vi "String - Convert Str (YYYY-mm-dd HHcMMcSS) to TimeStamp.vi"(11 "YYYY-mm-dd HH:MM:SS (String)":string="2014-09-24 13:30:59") -> (2 "time stamp":timestamp format="%<%I:%M:%S%3u %p\n%x>T", 3 "YYYY-mm-dd HH:MM:SS (String)":string)   [LabVIEW 2013]
uses:
  <vilib>/Utility/miscctls.llb/LVDateTimeRec.ctl
panel:
  out ".fractional second":string
  out "SS":string
  out "MM":string
  out "HH":string
  out "dd":string
  out "mm":string
  out "YYYY":string
  out "YYYY-mm-dd":string
  out "HH:MM:SS":string
  out "Array":string[](array[string])
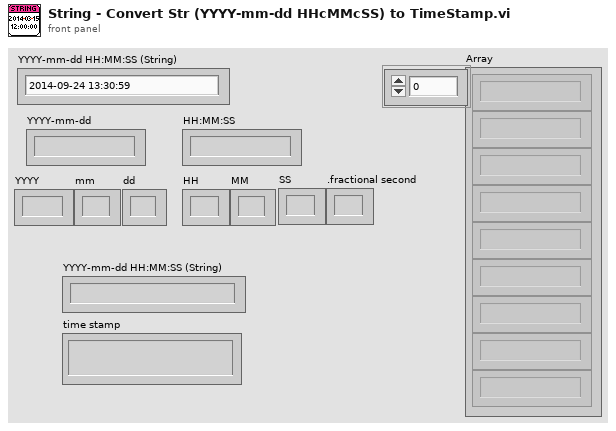
[diagram p1: front panel]
types:
  T1 = typedef "LVDateTimeRec.ctl" = cluster{"fractional second":dbl, "second":i32, "minute":i32, "hour":i32, "day of month":i32, "month":i32, "year":i32, "day of week":i32, "day of year":i32, "DST":i32}
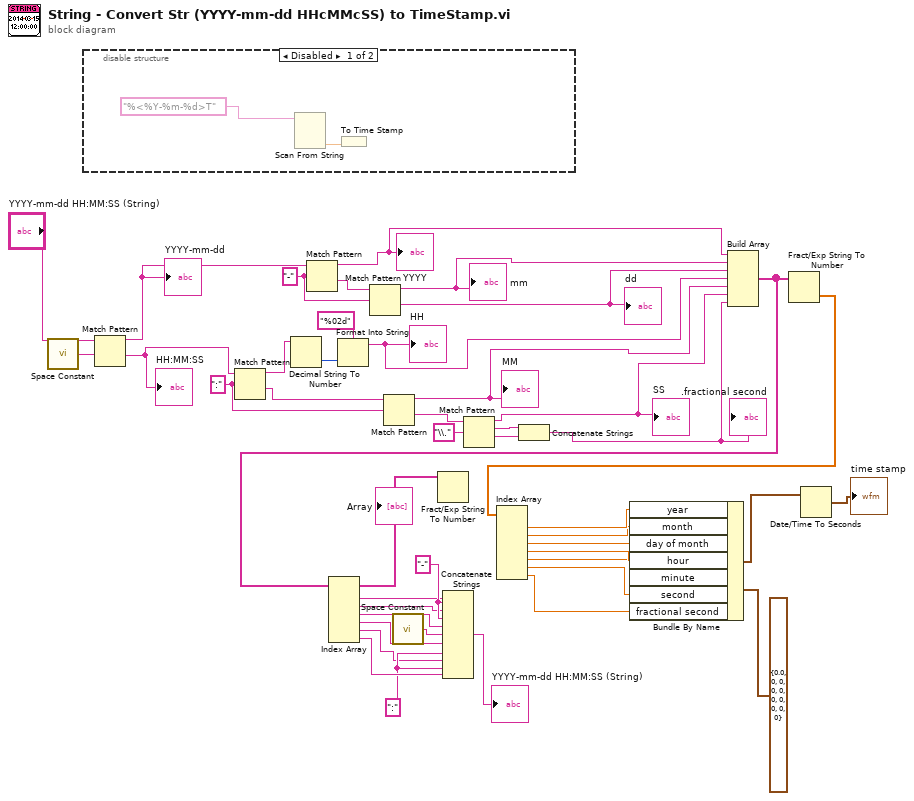
[diagram p0: block diagram]
diagram:
  w18 = ":" ("regular expression")
  w22 = "-" ("regular expression")
  w42 = ":"
  w38 = "-"
  n1 = call <vilib>:"Space Constant.vi"() -> ("String"=w24:string)
  n2 = disable-structure shown="Disabled" {
    frame Disabled {
      n3 = Scan From String(input string="%<%Y-%m-%d>T") -> (output 1=w45:dbl)  [unwired: 4 in, 3 out]
      n4 = To Time Stamp(1:w45) -> ()  [unwired: 1 out]
    }
    frame Enabled {
    }
  }
  n5 = Match Pattern(string="YYYY-mm-dd HH:MM:SS (String)", regular expression=w24) -> (before substring=w23:string, after substring=w20:string)  [unwired: 1 in, 2 out]
  "HH:MM:SS" <- w20
  "YYYY-mm-dd" <- w23
  n6 = Match Pattern(string=w20, regular expression=w18) -> (before substring=w3:string, after substring=w19:string)  [unwired: 1 in, 2 out]
  n7 = Decimal String To Number(string=w3) -> (number=w2:i32)  [unwired: 2 in, 1 out]
  n8 = Match Pattern(string=w23, regular expression=w22) -> (before substring=w17:string, after substring=w21:string)  [unwired: 1 in, 2 out]
  "YYYY" <- w17
  n9 = Format Into String(format string="%02d", w2) -> (resulting string=w1:string)  [unwired: 2 in, 1 out]
  "HH" <- w1
  n10 = Match Pattern(string=w21, regular expression=w22) -> (before substring=w16:string, after substring=w15:string)  [unwired: 1 in, 2 out]
  "mm" <- w16
  "dd" <- w15
  n11 = Match Pattern(string=w19, regular expression=w18) -> (before substring=w14:string, after substring=w11:string)  [unwired: 1 in, 2 out]
  "MM" <- w14
  n12 = call <vilib>:"Space Constant.vi"() -> ("String"=w35:string)
  n13 = Match Pattern(string=w11, regular expression="\\.") -> (before substring=w9:string, match substring=w7:string, after substring=w6:string)  [unwired: 1 in, 1 out]
  "SS" <- w9
  n14 = Concatenate Strings(w7, w6) -> (w5:string)
  ".fractional second" <- w5
  n15 = Build Array(w17, w16, w15, w1, w14, w9, w5) -> (w12:string[])
  "Array" <- w12
  n16 = Index Array(array=w12) -> (element #1=w36:string, element #2=w37:string, element #3=w39:string, element #4=w40:string, element #5=w41:string, element #6=w43:string)  [unwired: 6 in]
  n17 = Fract/Exp String To Number(string=w12) -> ()  [unwired: 3 in, 2 out]
  n18 = Concatenate Strings(w36, w38, w37, w38, w39, w35, w40, w42, w41, w42, w43) -> (→"YYYY-mm-dd HH:MM:SS (String)":string)
  n19 = Fract/Exp String To Number(string=w12) -> (number=w13:dbl[])  [unwired: 3 in, 1 out]
  n20 = Index Array(array=w13) -> (element #1=w33:dbl, element #2=w32:dbl, element #3=w31:dbl, element #4=w30:dbl, element #5=w29:dbl, element #6=w28:dbl, element #7=w8:dbl)  [unwired: 7 in]
  n21 = Bundle By Name(cluster=T1 {"fractional second"=0.0, "second"=0, "minute"=0, "hour"=0, "day of month"=0, "month"=0, "year"=0, "day of week"=0, "day of year"=0, "DST"=0} ("date time rec"), "year"=w33, "month"=w32, "day of month"=w31, "hour"=w30, "minute"=w29, "second"=w28, "fractional second"=w8) -> (w26:T1)
  n22 = Date/Time To Seconds(2:w26) -> (0:→"time stamp":timestamp)  [unwired: 1 in]
